vi "Create Thread Manager.vi"(7 "framework options":T1, 8 "error in (no error)":errorcluster, 9 "Public Threads":refnum<class "Thread.lvclass">[](array[class]), 10 "Private Threads":refnum<class "Thread.lvclass">[](array[class]), 11 "Framework in":refnum<class "Framework.lvclass">) -> (0 "error out":errorcluster, 3 "Framework out":refnum<class "Framework.lvclass">)   [LabVIEW 2017, in "DSF Core.lvlib" / "Framework.lvclass"]
uses:
  Framework.lvclass
  Thread/Thread.lvclass
  Framework Options.ctl
  Typedefs/DSF FIFO Options.ctl
  Thread/Thread Options.ctl
  Typedefs/DSF Plugin Options.ctl
  Typedefs/DSF Performance Options.ctl
  Framework.lvclass/Framework.ctl
  Thread Manager/Thread Manager.lvclass
  DSF Core.lvlib
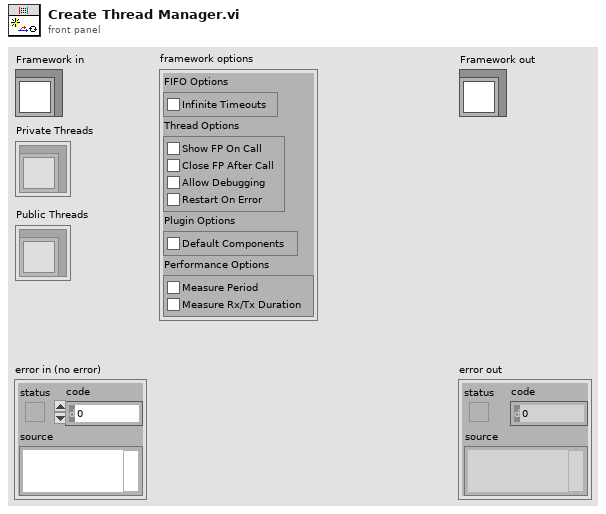
[diagram p1: front panel]
types:
  T1 = typedef "DSF Core.lvlib/Framework.lvclass/Framework Options.ctl" = cluster{"FIFO Options":T2, "Thread Options":T3, "Plugin Options":T4, "Performance Options":T5}
  T2 = typedef "DSF Core.lvlib/Framework.lvclass/DSF FIFO Options.ctl" = cluster{"Infinite Timeouts":bool}
  T3 = typedef "DSF Core.lvlib/Thread.lvclass/Thread Options.ctl" = cluster{"Show FP On Call":bool, "Close FP After Call":bool, "Allow Debugging":bool, "Restart On Error":bool}
  T4 = typedef "DSF Core.lvlib/Framework.lvclass/DSF Plugin Options.ctl" = cluster{"Default Components":bool}
  T5 = typedef "DSF Core.lvlib/DSF Performance Options.ctl" = cluster{"Measure Period":bool, "Measure Rx/Tx Duration":bool}
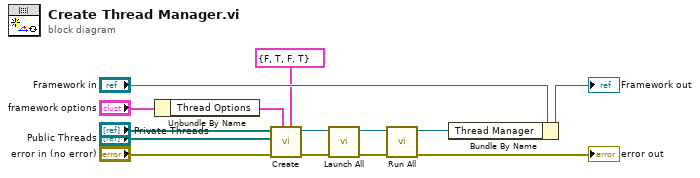
[diagram p0: block diagram]
diagram:
  n1 = Unbundle By Name("framework options") -> ("Thread Options"=w6:T3)
  n2 = call "Create.vi"("private thread options"=T3 {"Show FP On Call"=FALSE, "Close FP After Call"=TRUE, "Allow Debugging"=FALSE, "Restart On Error"=TRUE}, "public thread options"=w6, "error in (no error)"="error in (no error)", "Public Threads"="Public Threads", "Private Threads"="Private Threads") -> ("error out"=w13:errorcluster, "Thread Manager"=w14:refnum<class "Thread Manager.lvclass">)  [unwired: 5 in]
  n3 = call "Launch All.vi"("error in (no error)"=w13, "Thread Manager in"=w14) -> ("error out"=w4:errorcluster, "Thread Manager out"=w5:refnum<class "Thread Manager.lvclass">)  [unwired: 8 in]
  n4 = call "Run All.vi"("error in (no error)"=w4, "Thread Manager in"=w5) -> ("error out"=→"error out":errorcluster, "Thread Manager out"=w3:refnum<class "Thread Manager.lvclass">)  [unwired: 8 in]
  n5 = Bundle By Name(cluster="Framework in", "Thread Manager"=w3) -> (→"Framework out":refnum<class "Framework.lvclass">)
